vi "ADC_Interval.ph.vi"(0 "Frequency selection":enum16{"Closest", "Next highest"}(ring), 2 "Sampling rate (Hz)":dbl=1000.0 min=0.0 max=100000.0 format="%^.2e", 3 "error in (no error)":errorcluster, 4 "number of channels":i32) -> (6 "Actual Sampling Rate (Hz)":dbl format="%.2f", 7 "Scan Interval":string, 9 "error out":errorcluster)   [LabVIEW 2010]
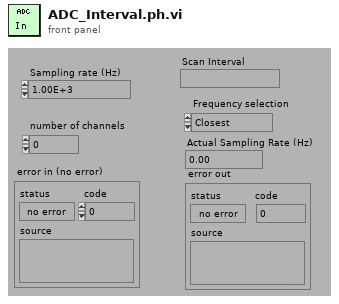
[diagram p1: front panel]
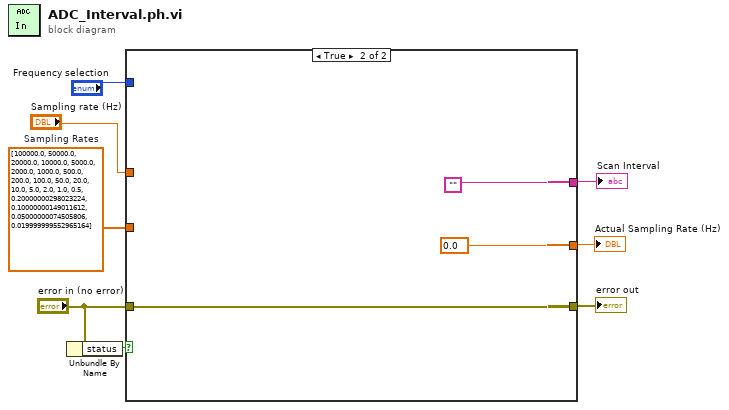
[diagram p0: block diagram]
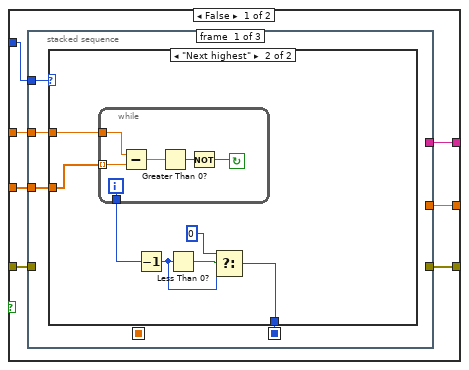
[diagram p2: hidden frame]
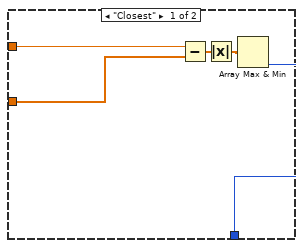
[diagram p3: hidden frame]
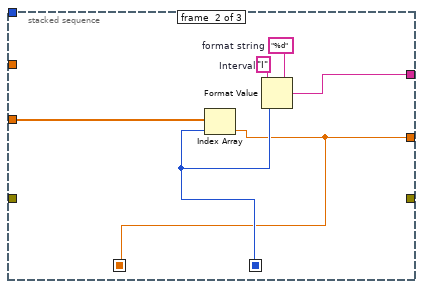
[diagram p4: hidden frame]
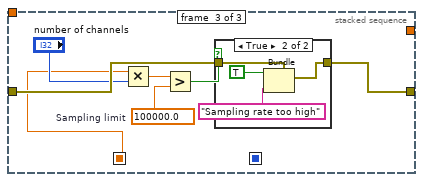
[diagram p5: hidden frame]
diagram:
  w1 = dbl[] [100000.0, 50000.0, 20000.0, 10000.0, 5000.0, 2000.0, 1000.0, 500.0, 200.0, 100.0, 50.0, 20.0, 10.0, 5.0, 2.0, 1.0, 0.5, 0.20000000298023224, 0.10000000149011612, 0.05000000074505806, 0.019999999552965164]  # Sampling Rates
  n1 = Unbundle By Name("error in (no error)") -> ("status"=w4:bool)
  n2 = case shown="True" w4 {
    tunnel: [w10 0.0] -> w7
    tunnel: [w9 ""] -> w8
    tunnel: [w14 w58] -> w6
    tunnel: "error in (no error)" -> [w15 w58]
    tunnel: "Frequency selection" -> [w13 _]
    tunnel: "Sampling rate (Hz)" -> [w12 _]
    tunnel: w1 -> [w11 _]
    frame False {
      n3 = stacked-sequence {
        seq-local: [w16 _ _] -> [_ w39 _]
        seq-local: [_ w38 _] -> [_ _ w44]
        tunnel: [_ _ w50] -> w14
        tunnel: w15 -> [_ _ w49]
        tunnel: w13 -> [w19 _ _]
        tunnel: w12 -> [w18 _ _]
        tunnel: w11 -> [w17 w41 _]
        tunnel: [_ w38 _] -> w10
        tunnel: [_ w40 _] -> w9
        frame #0 {
          n4 = case shown="\"Next highest\"" w19 {
            tunnel: w18 -> [w22 w31]
            tunnel: w17 -> [w21 w30]
            tunnel: [w20 w25] -> w16
            frame "Closest" {
              n5 = Subtract(x=w22, y=w21) -> (x-y=w24:dbl[])
              n6 = Absolute Value(x=w24) -> (abs(x)=w23:dbl[])
              n7 = Array Max & Min(array=w23) -> (min index (indices)=w20:i32)  [unwired: 3 out]
            }
            frame "Next highest" {
              n8 = while {
                tunnel: [w32] -> w29
                tunnel: w30 -> [w36] mode=indexing
                tunnel: w31 -> [w37]
                i -> [w32]
                stop <- w33 continue-if-true
                n9 = Subtract(x=w37, y=w36) -> (x-y=w35:dbl)
                n10 = Greater Than 0?(x=w35) -> (x > 0?=w34:bool)
                n11 = Not(x=w34) -> (.not. x?=w33:bool)
              }
              n12 = Decrement(x=w29) -> (x-1=w26:i32)
              n13 = Less Than 0?(x=w26) -> (x < 0?=w28:bool)
              n14 = Select(t=0, s=w28, f=w26) -> (s? t:f=w25:i32)
            }
          }
        }
        frame #1 {
          w42 = "%d"  # format string
          w43 = "I"  # Interval
          n15 = Index Array(array=w41, index=w39) -> (element=w38:dbl)
          n16 = Format Value(string ("")=w43, format string=w42, value (0)=w39) -> (output string=w40:string)
        }
        frame #2 {
          w47 = 100000.0  # Sampling limit
          n17 = Multiply(x=w44, y="number of channels") -> (x*y=w46:dbl)
          n18 = Greater?(x=w46, y=w47) -> (0:w48:bool)
          n19 = case shown="True" w48 {
            tunnel: w49 -> [w51 w54]
            tunnel: [w51 w55] -> w50
            frame False {
            }
            frame True {
              n20 = Bundle(cluster=w54, "status"=TRUE, "source"="Sampling rate too high") -> (w55:errorcluster)  [unwired: 1 out]
            }
          }
        }
      }
    }
    frame True {
    }
  }
  "Scan Interval" <- w8
  "Actual Sampling Rate (Hz)" <- w7
  "error out" <- w6
